vi "GetNormalizedColors.vi"(8 "error in (no error)":errorcluster, 11 "ColorSensorDevRef":T1={"I2CDevRef"={"DevStatus"={"status"=FALSE, "code"=0, "source"=""}, "Device Address"=0, "Handle"=0, "I2C Bus"=enum."Invalid"}} {"I2CDevRef"."Device Address" format="%.0x"}) -> (0 "error out":errorcluster, 2 "Normalized Colors":T4, 3 "ColorSensorDevRef out":T1={"I2CDevRef"={"DevStatus"={"status"=FALSE, "code"=0, "source"=""}, "Device Address"=0, "Handle"=0, "I2C Bus"=enum."Invalid"}} {"I2CDevRef"."Device Address" format="%.0x"})   [LabVIEW 2018, in "ColorSensor.lvlib"]
uses:
  ColorSensor.lvlib
  TypeDef/ColorSensorDevRef.ctl
  <vilib>/Rock Robotics/WPI/I2C/WPI_I2CDevRef.ctl
  <vilib>/Rock Robotics/SystemInterfaces/i2clib/i2c_bus.ctl
  TypeDef/NormColorValues.ctl
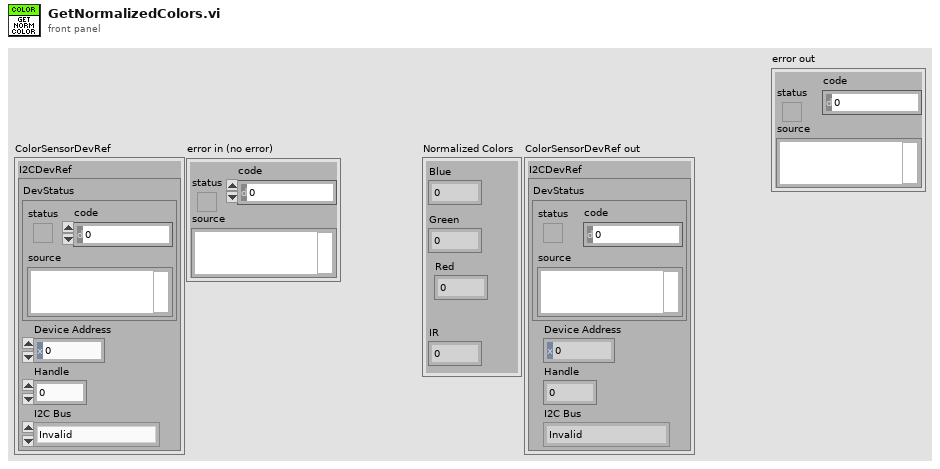
[diagram p1: front panel]
types:
  T1 = typedef "ColorSensor.lvlib/ColorSensorDevRef.ctl" = cluster{"I2CDevRef":T2}
  T2 = typedef "WPI_I2CDevRef.ctl" = cluster{"DevStatus":errorcluster, "Device Address":u8, "Handle":i32, "I2C Bus":T3}
  T3 = typedef "i2c_bus.ctl" = enum16{"I2C On-Board", "I2C MXP", "Invalid"}
  T4 = typedef "ColorSensor.lvlib/NormColorValues.ctl" = cluster{"Blue":dbl, "Green":dbl, "Red":dbl, "IR":dbl}
  T5 = typedef "ColorSensor.lvlib/ColorValues.ctl" = cluster{"IR":u32, "Green":u32, "Blue":u32, "Red":u32}
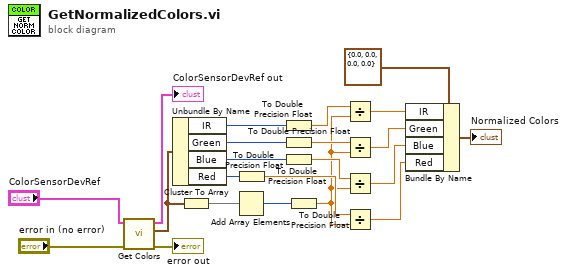
[diagram p0: block diagram]
diagram:
  n1 = call "Get Colors.vi"("error in (no error)"="error in (no error)", "ColorSensorDevRef"="ColorSensorDevRef") -> ("error out"=→"error out":errorcluster, "Color Values"=w19:T5, "ColorSensorDevRef out"=→"ColorSensorDevRef out":T1)  [unwired: 7 in]
  n2 = Unbundle By Name(w19) -> ("IR"=w17:u32, "Green"=w16:u32, "Blue"=w15:u32, "Red"=w14:u32)
  n3 = Cluster To Array(cluster=w19) -> (array=w20:u32[])
  n4 = Add Array Elements(numeric array=w20) -> (sum=w18:u32)
  n5 = To Double Precision Float(number=w14) -> (double precision float=w10:dbl)
  n6 = To Double Precision Float(number=w17) -> (double precision float=w13:dbl)
  n7 = To Double Precision Float(number=w16) -> (double precision float=w12:dbl)
  n8 = To Double Precision Float(number=w15) -> (double precision float=w11:dbl)
  n9 = To Double Precision Float(number=w18) -> (double precision float=w9:dbl)
  n10 = Divide(x=w13, y=w9) -> (x/y=w7:dbl)
  n11 = Divide(x=w12, y=w9) -> (x/y=w6:dbl)
  n12 = Divide(x=w11, y=w9) -> (x/y=w5:dbl)
  n13 = Divide(x=w10, y=w9) -> (x/y=w4:dbl)
  n14 = Bundle By Name(cluster=T4 {"Blue"=0.0, "Green"=0.0, "Red"=0.0, "IR"=0.0} ("NormColorValues"), "IR"=w7, "Green"=w6, "Blue"=w5, "Red"=w4) -> (→"Normalized Colors":T4)
